vi "Cooler OFF.vi"(8 "error in (no error)":errorcluster, 11 "Cooler in":refnum<class "Cooler.lvclass">) -> (0 "error out":errorcluster, 3 "Cooler out":refnum<class "Cooler.lvclass">)   [LabVIEW 2018, in "Cooler.lvclass"]
uses:
  Cooler.lvclass
  Cooler.lvclass/Cooler.ctl
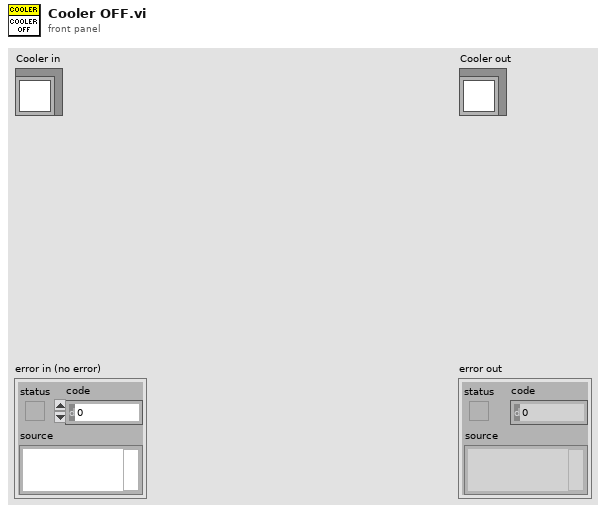
[diagram p1: front panel]
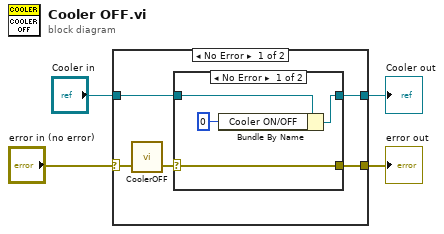
[diagram p0: block diagram]
diagram:
  n1 = case shown="No Error" "error in (no error)" {
    selector: "error in (no error)" -> [w9 w17]
    tunnel: [w7 w17] -> w2
    tunnel: [w5 w16] -> w3
    tunnel: "Cooler in" -> [w6 w16]
    frame No Error {
      n2 = call <userlib>:"CoolerOFF.vi"("error in (no error)"=w9) -> ("error out"=w8:errorcluster)  [unwired: 1 in, 1 out]
      n3 = case shown="No Error" w8 {
        selector: w8 -> [w13 w14]
        tunnel: [w13 w14] -> w7
        tunnel: w6 -> [w12 w15]
        tunnel: [w11 w15] -> w5
        frame No Error {
          n4 = Bundle By Name(cluster=w12, "Cooler ON/OFF"=u8 0) -> (w11:refnum<class "Cooler.lvclass">)
        }
        frame Error {
        }
      }
    }
    frame Error {
    }
  }
  "error out" <- w2
  "Cooler out" <- w3
